vi "SMU.GetConfiguration.vi"(8 "error in (no error)":errorcluster, 11 "SMU":refnum<class "SMU.lvclass">) -> (0 "error out":errorcluster, 2 "Configuration":T1, 3 "SMU out":refnum<class "SMU.lvclass">)   [LabVIEW 2019, in "SMU.lvclass"]
uses:
  SMU.lvclass
  Typedefs/Configuration--Cluster.ctl
  SMU.lvclass/SMU.ctl
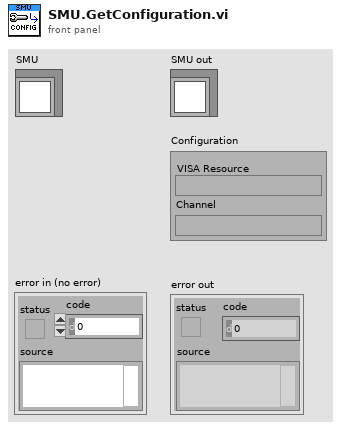
[diagram p1: front panel]
types:
  T1 = typedef "SMU.lvclass/Configuration--Cluster.ctl" = cluster{"VISA Resource":string, "Channel":string}
  T2 = typedef "SMU.lvclass/PrivateData--Ref.ctl" = refnum<data-value>
  T3 = typedef "SMU.lvclass/PrivateData--Cluster.ctl" = cluster{"Configuration":T1}
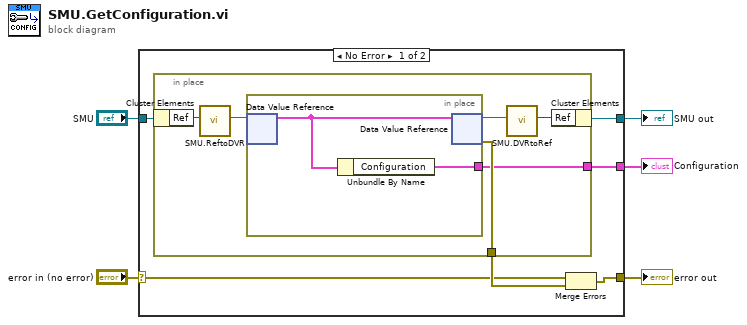
[diagram p0: block diagram]
diagram:
  n1 = case shown="No Error" "error in (no error)" {
    selector: "error in (no error)" -> [w7 w20]
    tunnel: "SMU" -> [w8 w21]
    tunnel: [w9 w20] -> w4
    tunnel: [w11 w21] -> w3
    tunnel: [w6 _] -> w1
    frame No Error {
      n2 = in-place {
        in-place-border: [w17] -> w10
        in-place-border: [w12] -> w6
        n3 = in-place-cluster #1(w8) -> ("Ref"=w16:u32)
        n4 = call "SMU.ReftoDVR.vi"("Ref"=w16) -> ("Ref"=w15:T2)  [unwired: 10 in]
        n5 = in-place {
          in-place-border: [w18] -> w12
          n6 = in-place-dvr #2(w15) -> (w19:T3)  [unwired: 1 out]
          n7 = Unbundle By Name(w19) -> ("Configuration"=w18:T1)
          n8 = in-place-dvr #2(w19) -> (w14:T2, w17:errorcluster)
        }
        n9 = call "SMU.DVRtoRef.vi"("Ref"=w14) -> ("Ref"=w13:u32)  [unwired: 10 in]
        n10 = in-place-cluster #1("Ref"=w13) -> (w11:refnum<class "SMU.lvclass">)
      }
      n11 = Merge Errors(w7, w10) -> (w9:errorcluster)
    }
    frame Error {
    }
  }
  "error out" <- w4
  "SMU out" <- w3
  "Configuration" <- w1
